vi "Actor Core.vi"(8 "error in":errorcluster, 11 "SolarSystems M266 in":refnum<class "SolarSystems M266.lvclass">) -> (0 "error out":errorcluster, 3 "Actor  out":refnum<class "Actor.lvclass">)   [LabVIEW 2014, in "SolarSystems M266.lvclass"]
uses:
  SolarSystems M266.lvclass
  Framework/Interfaces/Viewable Actor/Viewable Actor.lvclass
  Framework/Hardware/ParameterDevice/ParameterDevice.lvclass
  Framework/Interfaces/Observable Actor/Observable Actor.lvclass
  <vilib>/ActorFramework/Actor/Actor.lvclass
  Framework/Hardware/Device/Device Messages/Connect Msg/Connect Msg.lvclass
panel:
  out "Stop":bool=TRUE
  in  "Select Filter Wheel":i32(ring)=1 items=["Filter Wheel 1", "Filter Wheel 2"]
  in  "Select mirror":i32(ring)=1 items=["Mirror 1", "Mirror 2"]
  out "Pixel calibration":dbl
  out "XY Graph":cluster{"Y":dbl[], "Y":dbl[]}[](graph)
  in  "Get calibration":bool
  in  "Pixel Index":i32
  in  "Pixel Width":dbl
  in  "Central WL":dbl
  in  "Pixel Count":i32
  in  "Central Pixel":i32
  out "?":i32
  in  "Grating count":bool
  out "Grating":i32
  in  "Get active grating":bool
  in  "Set active grating":bool
  out "Max WL":dbl
  out "Min WL":dbl
  out "Grooves":i32
  in  "Grating":i32(ring) items=["Grating 1", "Grating 2", "Grating 3", "Grating 4"]
  in  "Reset active grating":bool
  out "Dispersion":dbl format="%.4f"
  out "Error":string
  out "Cur. state":i32(ring) items=["Unknown", "Open", "Close"]
  in  "Set shutter state":bool
  in  "Select shutter state":u32(ring) items=["Open", "Close"]
  out "Cur. filter":i32(ring) items=["Filter1", "Filter2", "Filter3", "Filter4", "Filter5", "Filter6", "Filter7", "Filter8"]
  in  "Set filter":bool
  in  "Select filter state":i32(ring) items=["Filter1", "Filter2", "Filter3", "Filter4", "Filter5", "Filter6", "Filter7", "Filter8"]
  out "Cur. mirror":i32(ring) items=["Undefined"=-1, "Axial port"=0, "Lateral port"=1]
  in  "Set mirror":bool
  in  "Select mirror state":i32(ring)=1 items=["Axial port"=1, "Lateral port"=2]
  in  "Reset":bool
  in  "Set slit width":bool
  out "Slit width":dbl format="%.2f"
  in  "Select slit":i32(ring) items=["Slit 1", "Slit 2", "Slit 3", "Slit 4"]
  in  "New slit width":dbl format="%.2f"
  in  "Set new WL":bool caption="Boolean"
  out "Cur WL":dbl format="%.2f"
  in  "New WL":dbl format="%.2f"
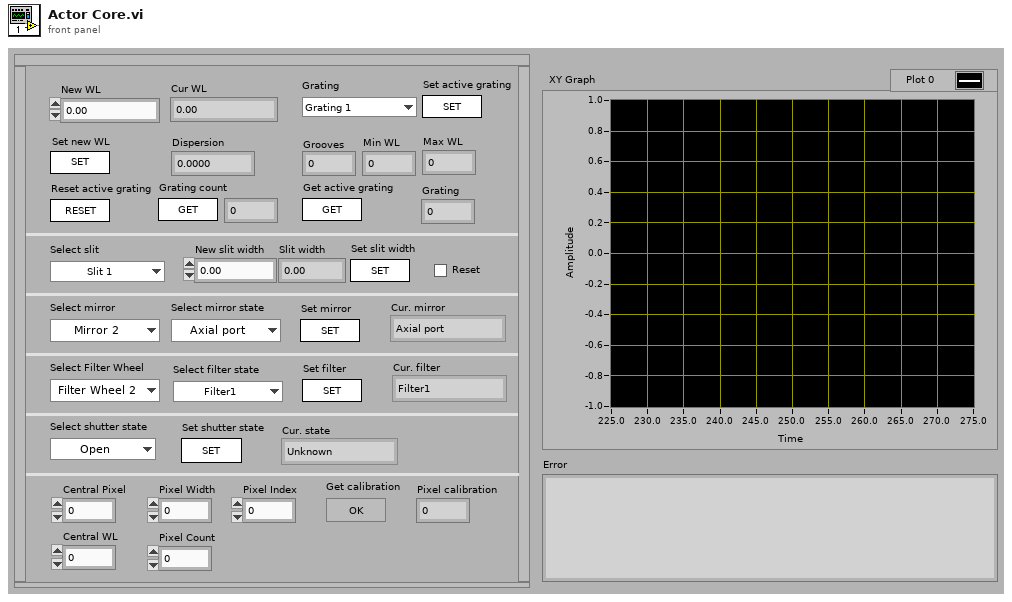
[diagram p1: front panel]
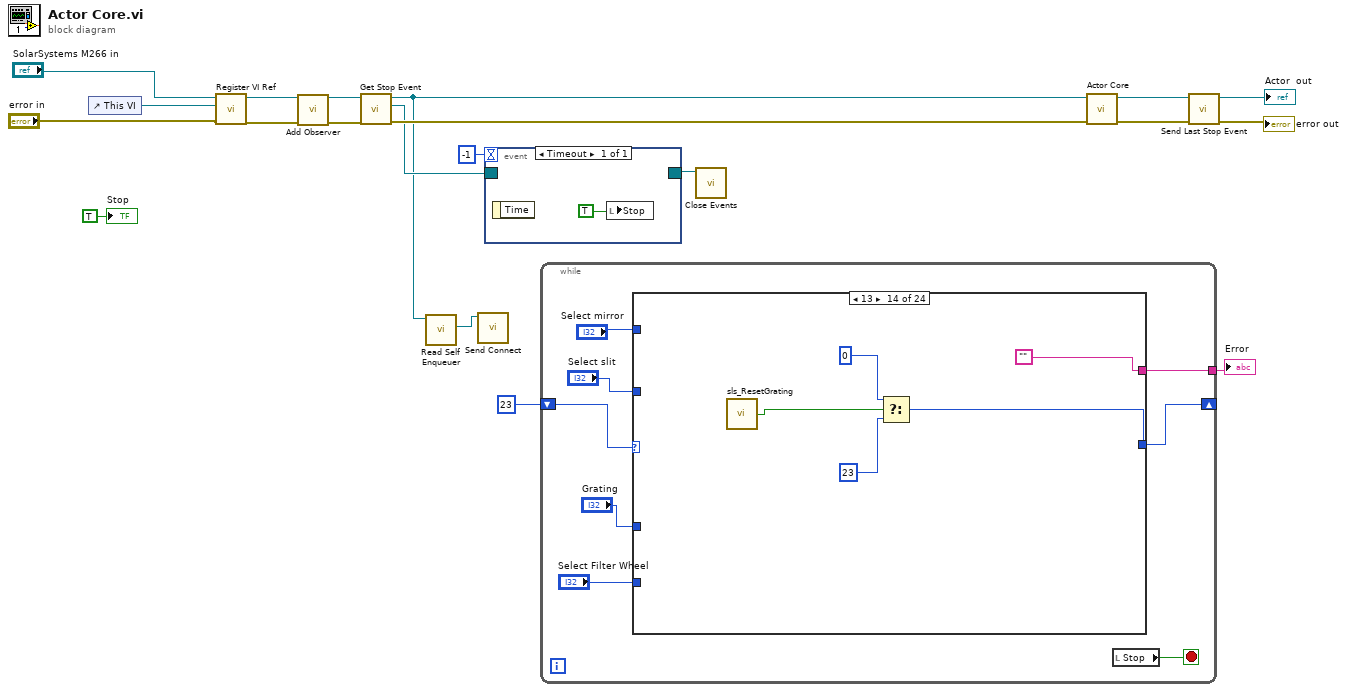
[diagram p0: block diagram]
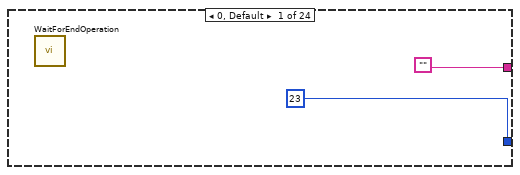
[diagram p2: hidden frame]
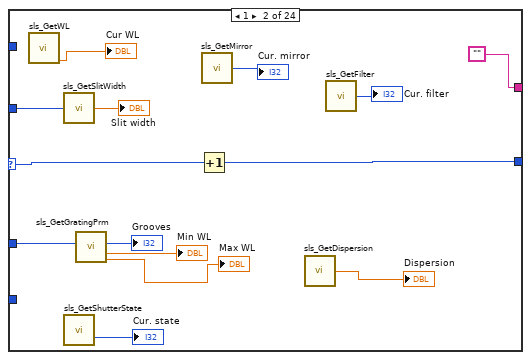
[diagram p3: hidden frame]
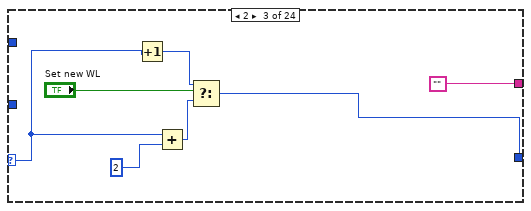
[diagram p4: hidden frame]
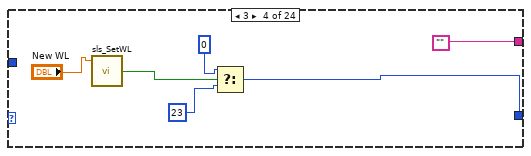
[diagram p5: hidden frame]
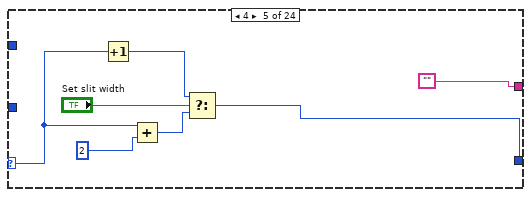
[diagram p6: hidden frame]
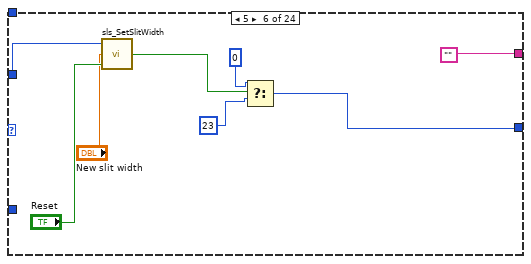
[diagram p7: hidden frame]
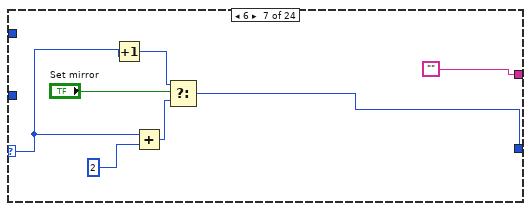
[diagram p8: hidden frame]
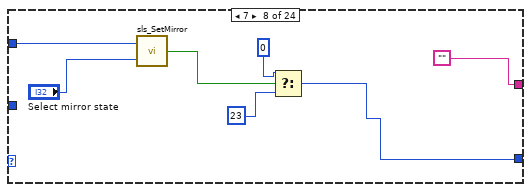
[diagram p9: hidden frame]
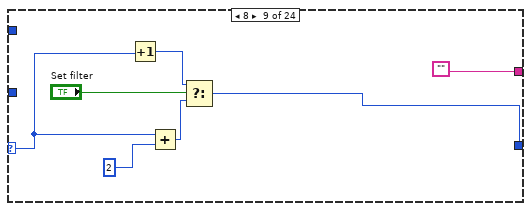
[diagram p10: hidden frame]
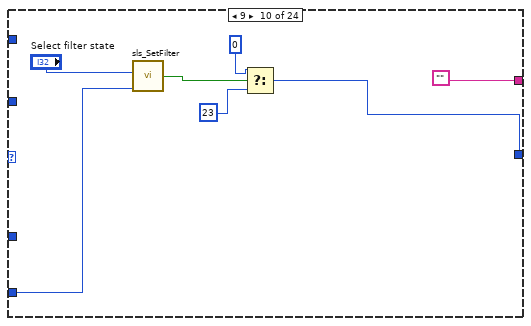
[diagram p11: hidden frame]
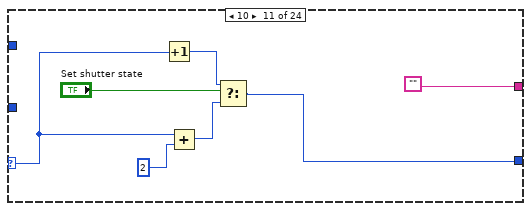
[diagram p12: hidden frame]
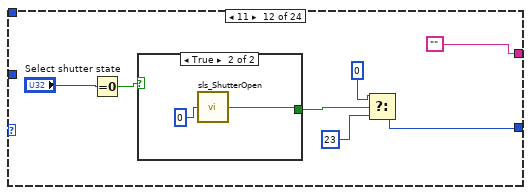
[diagram p13: hidden frame]
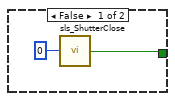
[diagram p14: hidden frame]
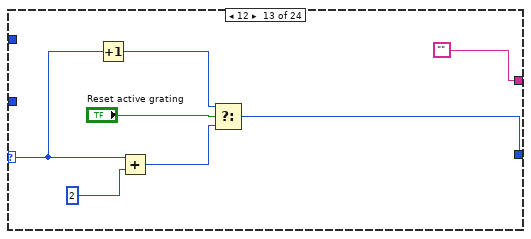
[diagram p15: hidden frame]
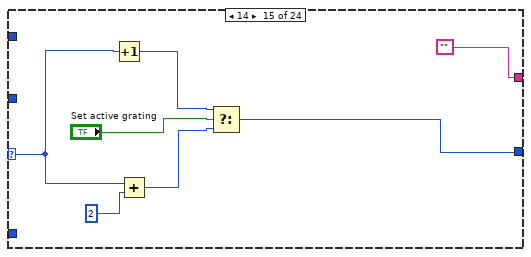
[diagram p16: hidden frame]
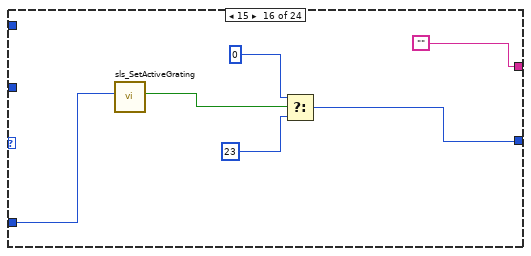
[diagram p17: hidden frame]
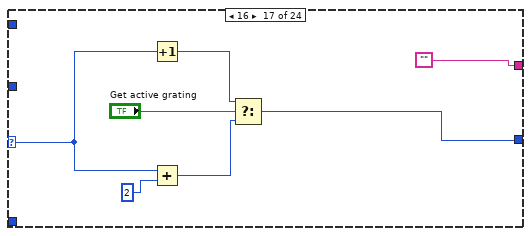
[diagram p18: hidden frame]
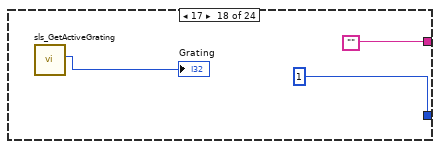
[diagram p19: hidden frame]
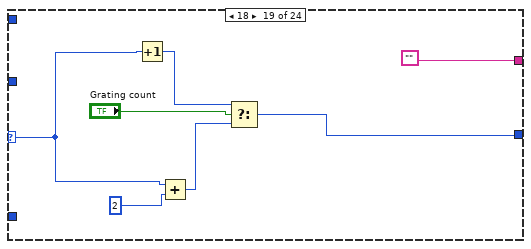
[diagram p20: hidden frame]
diagram:
  n1 = control-ref of="This VI"() -> (w12:refnum<vi>)
  n2 = call "Register VI Ref.vi"("error in (no error)"="error in", "VI ref"=w12, "Viewable Actor in"="SolarSystems M266 in") -> ("error out"=w14:errorcluster, "Viewable Actor out"=w13:refnum<class "SolarSystems M266.lvclass">)  [unwired: 7 in]
  n3 = call-dynamic "Add Observer.vi"("error in (no error)"=w14, "Observable Actor in"=w13) -> ("error out"=w19:errorcluster, "Observable Actor out"=w18:refnum<class "SolarSystems M266.lvclass">)  [unwired: 7 in, 1 out]
  n4 = call-dynamic "Get Stop Event.vi"("error in (no error)"=w19, "Observable Actor in"=w18) -> ("error out"=w17:errorcluster, "Events"=w5:refnum<event-registration>, "Observable Actor out"=w2:refnum<class "SolarSystems M266.lvclass">)  [unwired: 7 in]
  n5 = call <vilib>:"Read Self Enqueuer.vi"("Actor"=w2) -> ("Self Enqueuer"=w1:refnum<class "Message Enqueuer.lvclass">)  [unwired: 10 in]
  n6 = call "Send Connect.vi"("Message Enqueuer"=w1) -> ()  [unwired: 9 in, 2 out]
  n7 = event shown="[0] Timeout" {
    selector: w5 -> [_]
    dyn-events: [_] -> w3
    timeout: -1 ("Numeric") -> [_]
    event Timeout {
      n8 = event-data() -> ()  [unwired: 1 in, 1 out]
      n9 = local write "Stop"(TRUE) -> ()
    }
  }
  n10 = while {
    shift-right: [w28] -> _
    shift-left: 23 -> [w27]
    tunnel: [w23] -> w20
    stop <- w22 stop-if-true
    n11 = case shown="13" w27 {
      selector: w27 -> [_ w44 w47 _ w60 _ w76 _ w90 _ w106 _ w125 _ w138 _ w150 _ w160 _ w169 _ _ _]
      tunnel: "Select slit" -> [_ w35 _ _ _ w67 _ _ _ _ _ _ _ _ _ _ _ _ _ _ _ _ _ _]
      tunnel: [23 w45 w51 w56 w61 w71 w75 w86 w89 w99 w103 w113 w121 w129 w133 w142 w146 1 w156 1 w166 w181 1 1] -> w28
      tunnel: "Grating" -> [_ w43 _ _ _ _ _ _ _ _ _ _ _ _ _ w140 _ _ _ _ _ _ _ _]
      tunnel: "Select mirror" -> [_ _ _ _ _ _ _ w82 _ _ _ _ _ _ _ _ _ _ _ _ _ _ _ _]
      tunnel: "Select Filter Wheel" -> [_ _ _ _ _ _ _ _ _ w96 _ _ _ _ _ _ _ _ _ _ _ _ _ _]
      tunnel: ["" "" "" "" "" "" "" "" "" "" "" "" "" "" "" "" "" "" "" "" "" "" "" w191] -> w23
      frame 0, Default {
        n12 = call "WaitForEndOperation.vi"() -> ()  [unwired: 1 out]
      }
      frame 1 {
        n13 = call "sls_GetWL.vi"() -> ("Current WL"=→"Cur WL":dbl)  [unwired: 10 in, 1 out]
        n14 = call "sls_GetSlitWidth.vi"("Select slit"=w35) -> ("Slit width"=→"Slit width":dbl)
        n15 = call "sls_GetShutterState.vi"() -> ("Shutter state"=→"Cur. state":i32)
        n16 = call "sls_GetGratingPrm.vi"("Index grating"=w43) -> ("Max WL"=→"Max WL":dbl, "Min WL"=→"Min WL":dbl, "Grooves"=→"Grooves":i32)  [unwired: 7 in, 1 out]
        n17 = Increment(x=w44) -> (x+1=w45:i32)
        n18 = call "sls_GetMirror.vi"() -> ("Mirror position"=→"Cur. mirror":i32)
        n19 = call "sls_GetDispersion.vi"() -> ("Dispersion"=→"Dispersion":dbl)
        n20 = call "sls_GetFilter.vi"() -> ("Filter State"=→"Cur. filter":i32)
      }
      frame 2 {
        n21 = Increment(x=w47) -> (x+1=w50:i32)
        n22 = Add(x=w47, y=2) -> (x+y=w48:i32)
        n23 = Select(t=w50, s="Set new WL", f=w48) -> (s? t:f=w51:i32)
      }
      frame 3 {
        n24 = call "sls_SetWL.vi"("WL"="New WL") -> ("Result"=w55:bool)  [unwired: 2 in]
        n25 = Select(t=0, s=w55, f=23) -> (s? t:f=w56:i32)
      }
      frame 4 {
        n26 = Increment(x=w60) -> (x+1=w64:i32)
        n27 = Add(x=w60, y=2) -> (x+y=w63:i32)
        n28 = Select(t=w64, s="Set slit width", f=w63) -> (s? t:f=w61:i32)
      }
      frame 5 {
        n29 = call "sls_SetSlitWidth.vi"("Reset"="Reset", "Slit width"="New slit width", "Select slit"=w67) -> ("Result"=w70:bool)
        n30 = Select(t=0, s=w70, f=23) -> (s? t:f=w71:i32)
      }
      frame 6 {
        n31 = Increment(x=w76) -> (x+1=w80:i32)
        n32 = Add(x=w76, y=2) -> (x+y=w78:i32)
        n33 = Select(t=w80, s="Set mirror", f=w78) -> (s? t:f=w75:i32)
      }
      frame 7 {
        n34 = call "sls_SetMirror.vi"("Select mirror state"="Select mirror state", "Select Mirror"=w82) -> ("Result"=w84:bool)
        n35 = Select(t=0, s=w84, f=23) -> (s? t:f=w86:i32)
      }
      frame 8 {
        n36 = Increment(x=w90) -> (x+1=w94:i32)
        n37 = Add(x=w90, y=2) -> (x+y=w92:i32)
        n38 = Select(t=w94, s="Set filter", f=w92) -> (s? t:f=w89:i32)
      }
      frame 9 {
        n39 = call "sls_SetFilter.vi"("Select filter state"="Select filter state", "Select filter Wheel"=w96) -> ("Result"=w98:bool)
        n40 = Select(t=0, s=w98, f=23) -> (s? t:f=w99:i32)
      }
      frame 10 {
        n41 = Increment(x=w106) -> (x+1=w108:i32)
        n42 = Add(x=w106, y=2) -> (x+y=w104:i32)
        n43 = Select(t=w108, s="Set shutter state", f=w104) -> (s? t:f=w103:i32)
      }
      frame 11 {
        n44 = Equal To 0?(x="Select shutter state") -> (x = 0?=w111:bool)
        n45 = case shown="True" w111 {
          tunnel: [w117 w119] -> w110
          frame False {
            n46 = call "sls_ShutterClose.vi"("Shutter"=0) -> ("Result"=w117:bool)
          }
          frame True {
            n47 = call "sls_ShutterOpen.vi"("Shutter"=0) -> ("Result"=w119:bool)
          }
        }
        n48 = Select(t=0, s=w110, f=23) -> (s? t:f=w113:i32)
      }
      frame 12 {
        n49 = Increment(x=w125) -> (x+1=w124:i32)
        n50 = Add(x=w125, y=2) -> (x+y=w123:i32)
        n51 = Select(t=w124, s="Reset active grating", f=w123) -> (s? t:f=w121:i32)
      }
      frame 13 {
        n52 = call "sls_ResetGrating.vi"() -> ("Boolean"=w128:bool)
        n53 = Select(t=0, s=w128, f=23) -> (s? t:f=w129:i32)
      }
      frame 14 {
        n54 = Increment(x=w138) -> (x+1=w136:i32)
        n55 = Add(x=w138, y=2) -> (x+y=w135:i32)
        n56 = Select(t=w136, s="Set active grating", f=w135) -> (s? t:f=w133:i32)
      }
      frame 15 {
        n57 = call "sls_SetActiveGrating.vi"("Grating"=w140) -> ("Boolean"=w141:bool)  [unwired: 10 in]
        n58 = Select(t=0, s=w141, f=23) -> (s? t:f=w142:i32)
      }
      frame 16 {
        n59 = Increment(x=w150) -> (x+1=w149:i32)
        n60 = Add(x=w150, y=2) -> (x+y=w148:i32)
        n61 = Select(t=w149, s="Get active grating", f=w148) -> (s? t:f=w146:i32)
      }
      frame 17 {
        n62 = call "sls_GetActiveGrating.vi"() -> ("Active grating"=→"Grating":i32)  [unwired: 11 in]
      }
      frame 18 {
        n63 = Increment(x=w160) -> (x+1=w158:i32)
        n64 = Add(x=w160, y=2) -> (x+y=w157:i32)
        n65 = Select(t=w158, s="Grating count", f=w157) -> (s? t:f=w156:i32)
      }
      frame 19 {
        n66 = call "sls_GetGratingCount.vi"() -> ("Grating count"=→"?":i32)  [unwired: 11 in]
      }
      frame 20 {
        n67 = Increment(x=w169) -> (x+1=w170:i32)
        n68 = Add(x=w169, y=2) -> (x+y=w168:i32)
        n69 = Select(t=w170, s="Get calibration", f=w168) -> (s? t:f=w166:i32)
      }
      frame 21 {
        n70 = call "sls_GetPxlCalibration.vi"("Central WL"="Central WL", "Pxl Width"="Pixel Width", "Pxl Ind"="Pixel Index", "Central Pxl"="Central Pixel") -> ("Pixel Calibration"=→"Pixel calibration":dbl, "Boolean"=w178:bool)  [unwired: 6 in]
        n71 = call "sls_GetCalibration.vi"("Central Wawelength"="Central WL", "Pixel Pitch"="Pixel Width", "Pixel Count"="Pixel Count", "Central Pixel"="Central Pixel") -> ("Waveform Graph"=w180:dbl[])  [unwired: 5 in, 1 out]
        n72 = Multiply(x=w180, y=0) -> (x*y=w185:dbl[])
        n73 = call "Convert to Dynamic Data"("Array"=w180) -> ("Dynamic Data Type"=w187:dynamicdata)  [unwired: 3 in]
        n74 = call "Convert to Dynamic Data2"("Array"=w185) -> ("Dynamic Data Type"=w184:dynamicdata)  [unwired: 3 in]
        n75 = call "Build XY Graph"("Y Input"=w184, "X Input"=w187) -> ("XY Graph"=→"XY Graph":cluster{"Y":dbl[], "Y":dbl[]}[])  [unwired: 3 in, 6 out]
        n76 = Select(t=0, s=w178, f=23) -> (s? t:f=w181:i32)
      }
      frame 22 {
      }
      frame 23 {
        n77 = call "sls_GetError.vi"() -> ("Error text"=w191:string)  [unwired: 1 in]
      }
    }
    n78 = local read "Stop"() -> (w22:bool)
  }
  "Error" <- w20
  n79 = call "Close Events.vi"("events"=w3) -> ()  [unwired: 11 in]
  n80 = call-parent "Actor Core.vi"("error in"=w17, "Actor in"=w2) -> ("error out"=w15:errorcluster, "Actor out"=w16:refnum<class "Actor.lvclass">)  [unwired: 8 in]
  n81 = call "Send Last Stop Event.vi"("error in (no error)"=w15, "Actor in"=w16) -> ("error out"=→"error out":errorcluster, "Actor  out"=→"Actor  out":refnum<class "Actor.lvclass">)  [unwired: 8 in]
  "Stop" <- TRUE ("Stop")
